vi "JIO_OnePannel_PhaseCali_Ken.vi"() -> ()   [LabVIEW 2023, in "JIO.lvlib"]
uses:
  JIO.lvlib
  FTDI/JIO/CLC_JIO_FTDI.lvlib
  R_S/R_S.lvlib
  Anritsu/Anritsu.lvlib
panel:
  in  "File_note":string
  out "error out":errorcluster
  out "Time(64-Steps)sec":dbl
  out "Phase":i32
  out "Channel":i32
  out "IC_No.":i32
  out "Chain":i32
  out "Power Sensor (dB)":dbl[](graph)
  in  "Waiting Time(ms)":u32=1000
  in  "error in":errorcluster
  in  "Ref_gain":i32
  in  "Ref_Phase":i32
  in  "Ref_Channel":i32
  in  "Ref_IC_":i32
  in  "Ref_Chain":i32
  in  "Channel_setting":T1
  # "JIO Phase Calibration for TMYTEK"
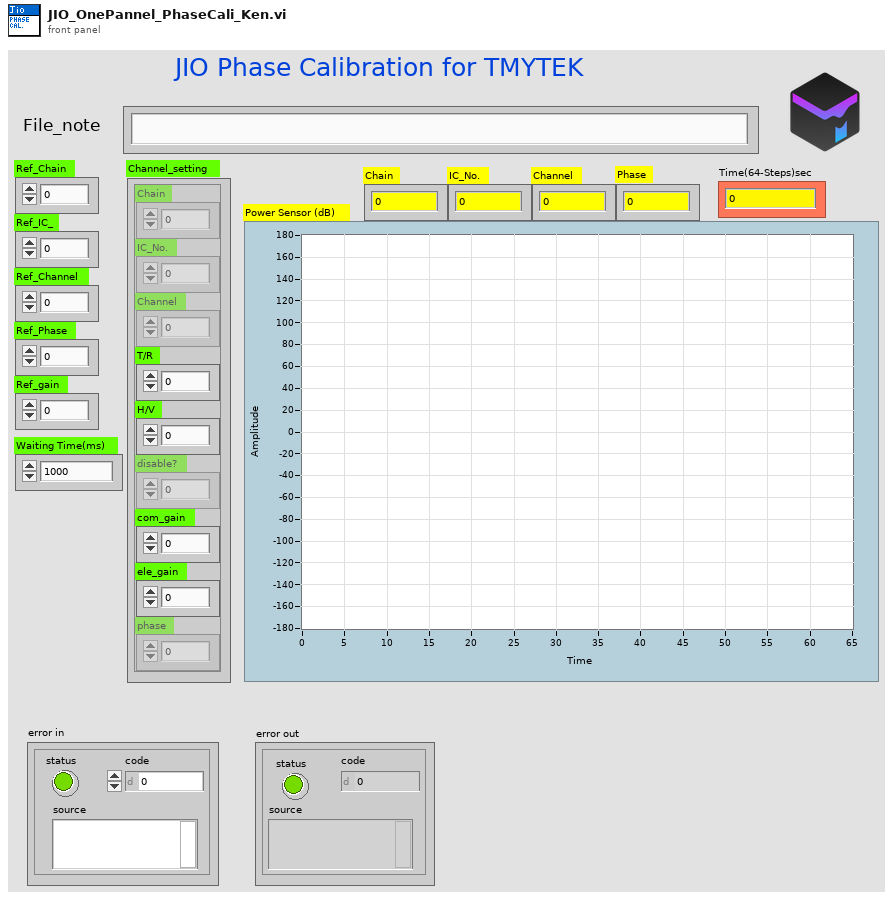
[diagram p1: front panel]
types:
  T1 = cluster{"Chain":i32, "IC_No.":i32, "Channel":i32, "T/R":i32, "H/V":i32, "disable?":i32, "com_gain":i32, "ele_gain":i32, "phase":i32}
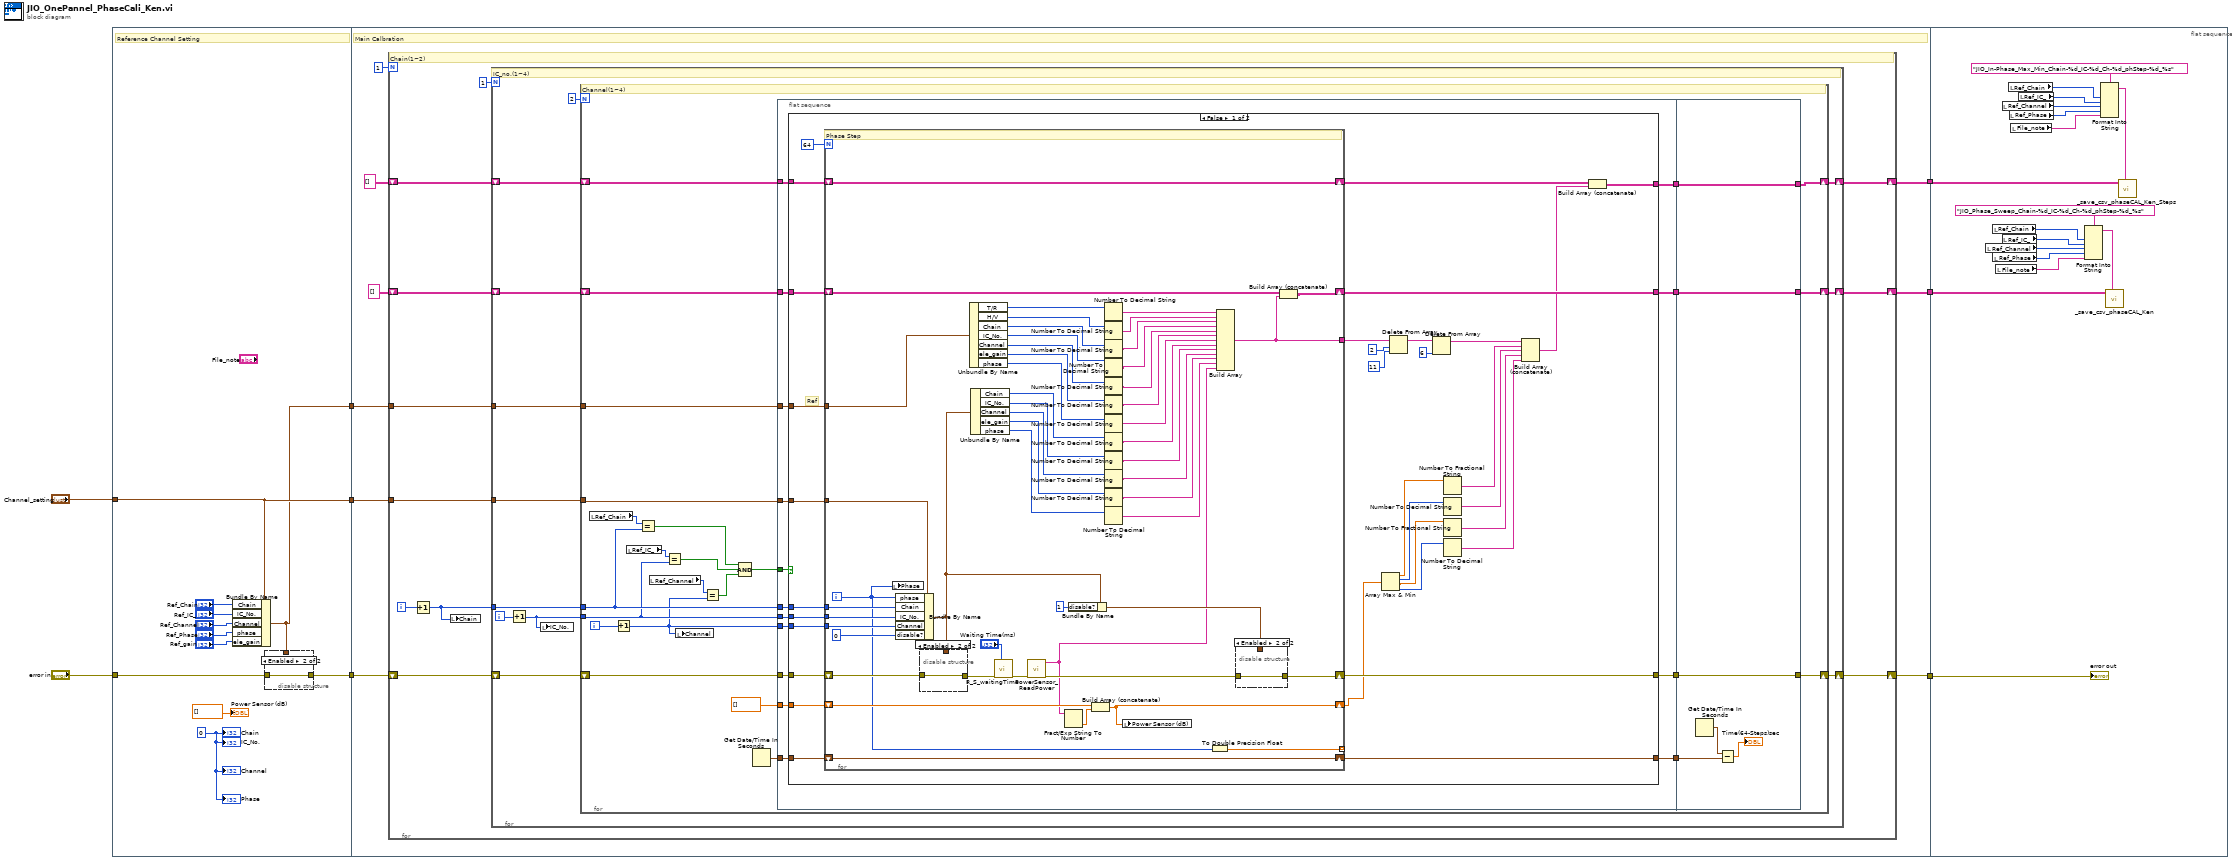
[diagram p0: block diagram]
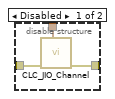
[diagram p2: hidden frame]
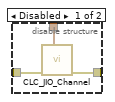
[diagram p3: hidden frame]
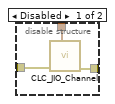
[diagram p4: hidden frame]
diagram:
  n1 = flat-sequence {
    tunnel: "Channel_setting" -> [w19]
    tunnel: [w19] -> w7
    tunnel: "error in" -> [w13]
    tunnel: [w12] -> w5
    tunnel: [w9] -> w4
    tunnel: w7 -> [w31]
    tunnel: w5 -> [w30]
    tunnel: w4 -> [w29]
    tunnel: [w27] -> w3
    tunnel: [w26] -> w2
    tunnel: [w24] -> w1
    tunnel: w3 -> [w212]
    tunnel: w2 -> [w211]
    tunnel: w1 -> [w198]
    frame #0 {
      w10 = 0 ("Chain")
      # "Reference Channel Setting"
      n2 = Bundle By Name(cluster=w19, "Chain"="Ref_Chain", "IC_No."="Ref_IC_", "Channel"="Ref_Channel", "phase"="Ref_Phase", "ele_gain"="Ref_gain") -> (w9:T1)
      n3 = disable-structure shown="Enabled" {
        disable-tunnel: w13 -> [w22 w23]
        disable-tunnel: [w21 w23] -> w12
        disable-tunnel: w9 -> [w20 _]
        frame Disabled {
          n4 = call "CLC_JIO_Channel.vi"("Channel_setting"=w20, "error in"=w22) -> ("error out"=w21:errorcluster)  [unwired: 8 in, 1 out]
        }
        frame Enabled {
        }
      }
      "Power Sensor (dB)" <- dbl[] [] ("Power Sensor (dB)")
      "Chain" <- w10
      "IC_No." <- w10
      "Channel" <- w10
      "Phase" <- w10
    }
    frame #1 {
      # "Main Calbration"
      n5 = for {
        N: 1 -> [_]
        tunnel: w31 -> [w42]
        shift-right: [w40] -> w27
        shift-left: w30 -> [w41]
        tunnel: w29 -> [w38]
        shift-right: [w36] -> w26
        shift-left: string[][] [] -> [w37]
        shift-right: [w34] -> w24
        shift-left: string[][] [] -> [w35]
        i -> [w39]
        # "Chain(1~2)"
        n6 = Increment(x=w39) -> (x+1=w33:i32)
        n7 = local write "Chain"(w33) -> ()
        n8 = for {
          N: 1 -> [_]
          tunnel: w42 -> [w54]
          tunnel: w33 -> [w53]
          shift-right: [w51] -> w40
          shift-left: w41 -> [w52]
          tunnel: w38 -> [w49]
          shift-right: [w47] -> w36
          shift-left: w37 -> [w48]
          shift-right: [w45] -> w34
          shift-left: w35 -> [w46]
          i -> [w50]
          # "IC_no.(1~4)"
          n9 = Increment(x=w50) -> (x+1=w44:i32)
          n10 = local write "IC_No."(w44) -> ()
          n11 = for {
            N: 2 -> [_]
            tunnel: w54 -> [w79]
            tunnel: w44 -> [w57]
            tunnel: w53 -> [w58]
            shift-right: [w70] -> w51
            shift-left: w52 -> [w80]
            tunnel: w49 -> [w68]
            shift-right: [w66] -> w47
            shift-left: w48 -> [w67]
            shift-right: [w59] -> w45
            shift-left: w46 -> [w61]
            i -> [w69]
            # "Channel(1~4)"
            n12 = local read "Ref_Chain"() -> (w78:i32)
            n13 = Increment(x=w69) -> (x+1=w56:i32)
            n14 = local read "Ref_IC_"() -> (w77:i32)
            n15 = Equal?(x=w78, y=w58) -> (x = y?=w75:bool)
            n16 = local read "Ref_Channel"() -> (w76:i32)
            n17 = Equal?(x=w77, y=w57) -> (x = y?=w74:bool)
            n18 = local write "Channel"(w56) -> ()
            n19 = Equal?(x=w76, y=w56) -> (x = y?=w73:bool)
            n20 = Compound Arithmetic op=AND(w75, w74, w73) -> (w72:bool)
            n21 = Get Date/Time In Seconds() -> (seconds since 1Jan1904=w65:timestamp)
            n22 = flat-sequence {
              tunnel: w80 -> [w95]
              tunnel: w79 -> [w94]
              tunnel: w58 -> [w93]
              tunnel: w57 -> [w92]
              tunnel: w72 -> [w91]
              tunnel: dbl[] [] ("Power Sensor (dB)") -> [w90]
              tunnel: w56 -> [w88]
              tunnel: w68 -> [w87]
              tunnel: w67 -> [w86]
              tunnel: w65 -> [w84]
              tunnel: [w89] -> w64
              tunnel: [w85] -> w63
              tunnel: [w83] -> w62
              tunnel: w61 -> [w82]
              tunnel: [w81] -> w60
              tunnel: [w194] -> w66
              tunnel: [w195] -> w70
              tunnel: w64 -> [w195]
              tunnel: w63 -> [w194]
              tunnel: w62 -> [w191]
              tunnel: w60 -> [w190]
              tunnel: [w190] -> w59
              frame #0 {
                n23 = case shown="False" w91 {
                  tunnel: w93 -> [w127 _]
                  tunnel: w92 -> [w126 _]
                  tunnel: w88 -> [w125 _]
                  tunnel: w95 -> [w124 w189]
                  tunnel: w94 -> [w123 _]
                  tunnel: [w121 w189] -> w89
                  tunnel: w90 -> [w120 _]
                  tunnel: w87 -> [w119 _]
                  tunnel: w86 -> [w118 w188]
                  tunnel: [w117 w188] -> w85
                  tunnel: w84 -> [w116 w187]
                  tunnel: [w115 w187] -> w83
                  tunnel: w82 -> [w99 w186]
                  tunnel: [w96 w186] -> w81
                  frame False {
                    # "Ref"
                    n24 = for {
                      N: 64 -> [_]
                      tunnel: w127 -> [w177]
                      tunnel: w126 -> [w176]
                      tunnel: w125 -> [w175]
                      tunnel: w123 -> [w161]
                      shift-right: [w168] -> w121
                      shift-left: w124 -> [w174]
                      shift-right: [w163] -> w114
                      shift-left: w120 -> [w165]
                      tunnel: w119 -> [w157]
                      shift-right: [w135] -> w117
                      shift-left: w118 -> [w134]
                      shift-right: [w132] -> w115
                      shift-left: w116 -> [w132]
                      tunnel: [w130] -> _ mode=indexing
                      tunnel: [w129] -> w113
                      shift-right: [w128] -> w98
                      shift-left: w99 -> [w128]
                      i -> [w131]
                      # "Phase Step"
                      n25 = local write "Phase"(w131) -> ()
                      n26 = Bundle By Name(cluster=w161, "phase"=w131, "Chain"=w177, "IC_No."=w176, "Channel"=w175, "disable?"=0) -> (w162:T1)
                      n27 = disable-structure shown="Enabled" {
                        disable-tunnel: w174 -> [w184 w185]
                        disable-tunnel: [w183 w185] -> w172
                        disable-tunnel: w162 -> [w182 _]
                        frame Disabled {
                          n28 = call "CLC_JIO_Channel.vi"("Channel_setting"=w182, "error in"=w184) -> ("error out"=w183:errorcluster)  [unwired: 8 in, 1 out]
                        }
                        frame Enabled {
                        }
                      }
                      n29 = Unbundle By Name(w157) -> ("T/R"=w160:i32, "H/V"=w159:i32, "Chain"=w158:i32, "IC_No."=w156:i32, "Channel"=w155:i32, "ele_gain"=w154:i32, "phase"=w153:i32)
                      n30 = Unbundle By Name(w162) -> ("Chain"=w152:i32, "IC_No."=w151:i32, "Channel"=w150:i32, "ele_gain"=w149:i32, "phase"=w148:i32)
                      n31 = call "R_S_waitingTime.vi"("Waiting Time(ms)"="Waiting Time(ms)", "error in"=w172) -> ("error out"=w167:errorcluster)  [unwired: 9 in]
                      n32 = call "PowerSensor_ReadPower.vi"("error in"=w167) -> ("error out"=w166:errorcluster, "Response"=w133:string)  [unwired: 9 in]
                      n33 = Fract/Exp String To Number(string=w133) -> (number=w164:dbl)  [unwired: 3 in, 1 out]
                      n34 = Bundle By Name(cluster=w162, "disable?"=1) -> (w169:T1)
                      n35 = Build Array (concatenate)(w165, w164) -> (w163:dbl[])
                      n36 = Number To Decimal String(number=w160) -> (decimal integer string=w147:string)  [unwired: 1 in]
                      n37 = Number To Decimal String(number=w159) -> (decimal integer string=w146:string)  [unwired: 1 in]
                      n38 = Number To Decimal String(number=w158) -> (decimal integer string=w145:string)  [unwired: 1 in]
                      n39 = Number To Decimal String(number=w156) -> (decimal integer string=w144:string)  [unwired: 1 in]
                      n40 = Number To Decimal String(number=w155) -> (decimal integer string=w143:string)  [unwired: 1 in]
                      n41 = Number To Decimal String(number=w154) -> (decimal integer string=w142:string)  [unwired: 1 in]
                      n42 = Number To Decimal String(number=w153) -> (decimal integer string=w141:string)  [unwired: 1 in]
                      n43 = Number To Decimal String(number=w152) -> (decimal integer string=w140:string)  [unwired: 1 in]
                      n44 = Number To Decimal String(number=w151) -> (decimal integer string=w139:string)  [unwired: 1 in]
                      n45 = Number To Decimal String(number=w150) -> (decimal integer string=w138:string)  [unwired: 1 in]
                      n46 = Number To Decimal String(number=w149) -> (decimal integer string=w137:string)  [unwired: 1 in]
                      n47 = Number To Decimal String(number=w148) -> (decimal integer string=w136:string)  [unwired: 1 in]
                      n48 = local write "Power Sensor (dB)"(w163) -> ()
                      n49 = To Double Precision Float(number=w131) -> (double precision float=w130:dbl)
                      n50 = Build Array(w147, w146, w145, w144, w143, w142, w141, w140, w139, w138, w137, w136, w133) -> (w129:string[])
                      n51 = disable-structure shown="Enabled" {
                        disable-tunnel: w169 -> [w180 _]
                        disable-tunnel: [w179 w181] -> w168
                        disable-tunnel: w166 -> [w178 w181]
                        frame Disabled {
                          n52 = call "CLC_JIO_Channel.vi"("Channel_setting"=w180, "error in"=w178) -> ("error out"=w179:errorcluster)  [unwired: 8 in, 1 out]
                        }
                        frame Enabled {
                        }
                      }
                      n53 = Build Array (concatenate)(w134, w129) -> (w135:string[][])
                    }
                    n54 = Array Max & Min(array=w114) -> (max value=w107:dbl, max index (indices)=w105:i32, min value=w104:dbl, min index (indices)=w103:i32)
                    n55 = Delete From Array(array=w113, length=2, index=11) -> (array with subset deleted=w110:string[])  [unwired: 1 out]
                    n56 = Delete From Array(array=w110, index=6) -> (array with subset deleted=w108:string[])  [unwired: 1 in, 1 out]
                    n57 = Number To Fractional String(number=w107) -> (F-format string=w106:string)  [unwired: 3 in]
                    n58 = Number To Decimal String(number=w105) -> (decimal integer string=w102:string)  [unwired: 1 in]
                    n59 = Number To Fractional String(number=w104) -> (F-format string=w101:string)  [unwired: 3 in]
                    n60 = Number To Decimal String(number=w103) -> (decimal integer string=w100:string)  [unwired: 1 in]
                    n61 = Build Array (concatenate)(w108, w106, w102, w101, w100) -> (w97:string[])
                    n62 = Build Array (concatenate)(w98, w97) -> (w96:string[][])
                  }
                  frame True {
                  }
                }
              }
              frame #1 {
                n63 = Get Date/Time In Seconds() -> (seconds since 1Jan1904=w192:timestamp)
                n64 = Subtract(x=w192, y=w191) -> (x-y=→"Time(64-Steps)sec":dbl)
              }
            }
          }
        }
      }
    }
    frame #2 {
      n65 = local read "Ref_Channel"() -> (w206:i32)
      n66 = local read "Ref_Chain"() -> (w208:i32)
      n67 = local read "Ref_Phase"() -> (w205:i32)
      n68 = local read "File_note"() -> (w197:string)
      n69 = local read "Ref_Channel"() -> (w203:i32)
      n70 = local read "Ref_IC_"() -> (w207:i32)
      n71 = local read "Ref_Chain"() -> (w201:i32)
      n72 = local read "Ref_Phase"() -> (w204:i32)
      n73 = local read "File_note"() -> (w196:string)
      n74 = local read "Ref_IC_"() -> (w202:i32)
      n75 = Format Into String(format string="JIO_Phase_Sweep_Chain-%d_IC-%d_Ch-%d_phStep-%d_%s", w208, w207, w206, w205, w197) -> (resulting string=w209:string)  [unwired: 2 in, 1 out]
      n76 = Format Into String(format string="JIO_In-Phase_Max_Min_Chain-%d_IC-%d_Ch-%d_phStep-%d_%s", w201, w202, w203, w204, w196) -> (resulting string=w200:string)  [unwired: 2 in, 1 out]
      n77 = call "_save_csv_phaseCAL_Ken.vi"("NoteName"=w209, "array in"=w211) -> ()  [unwired: 10 in]
      n78 = call "_save_csv_phaseCAL_Ken_Steps.vi"("NoteName"=w200, "array in"=w198) -> ()  [unwired: 10 in]
      "error out" <- w212
    }
  }
